vi "SUB_Chk_SWVer_MCS.vi"() -> (0 "SwVer_MCS":string, 1 "OK ?":bool)   [LabVIEW 2011]
uses:
  Instance           5 25Saved   SUB_Chk_SWVer_MCS .vi
  Instance           7 25Saved   SUB_Chk_SWVer_MCS .vi
  data/MCSDLL.dll
panel:
  out "Current Software Version":string
  out "UUT Model Type":string
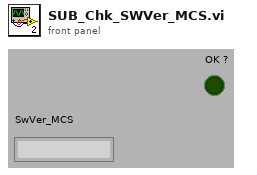
[diagram p1: front panel]
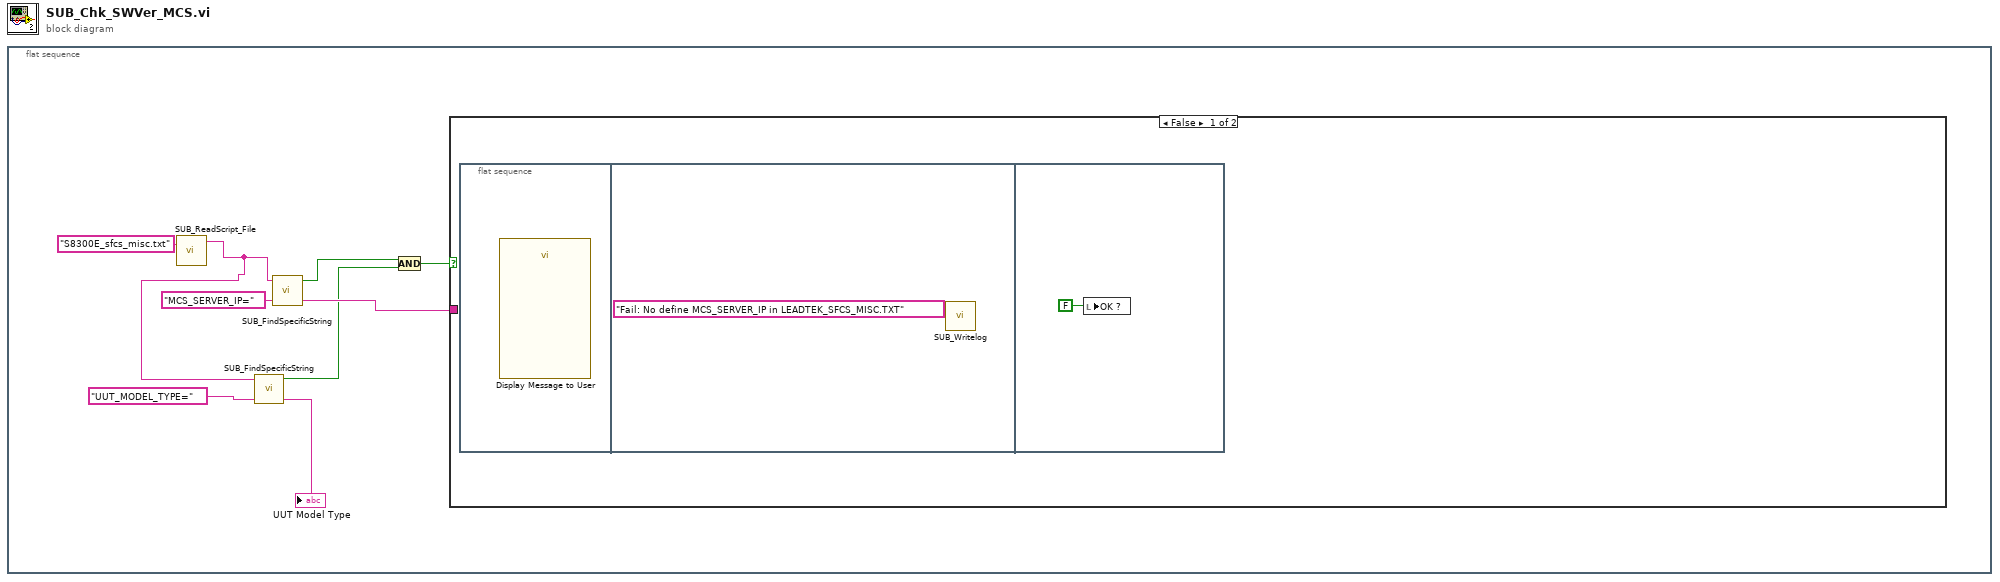
[diagram p0: block diagram]
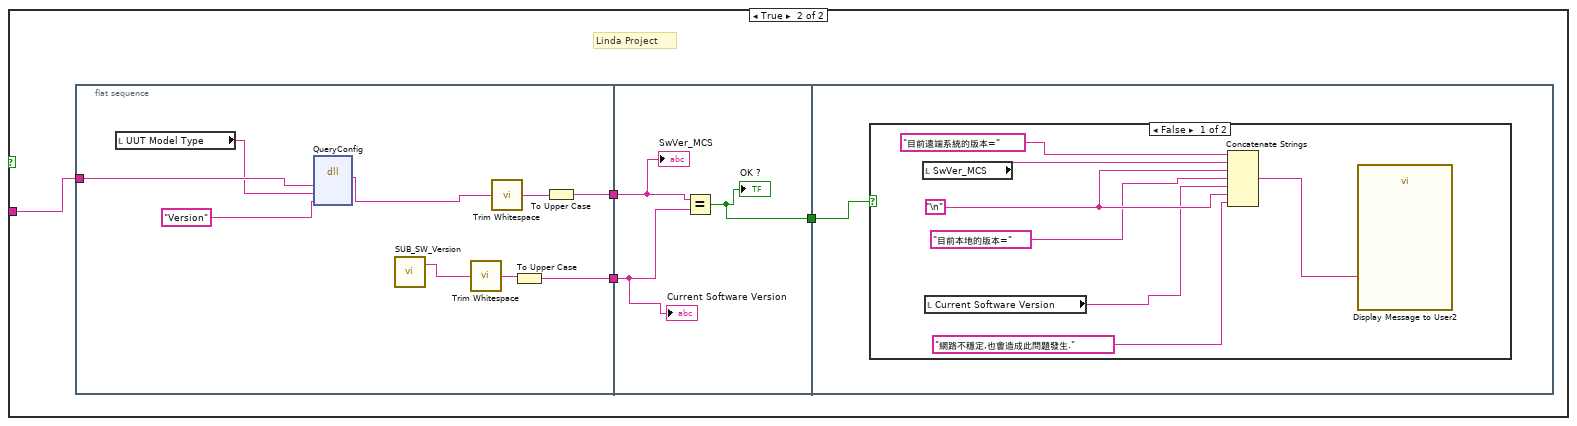
[diagram p2: hidden frame]
diagram:
  n1 = flat-sequence {
    frame #0 {
      n2 = call "SUB_ReadScript_File.vi"("Script FileName"="S8300E_sfcs_misc.txt") -> ("text"=w5:string)  [unwired: 1 in, 2 out]
      n3 = call "SUB_FindSpecificString.vi"("Find this String"="UUT_MODEL_TYPE=", "String data"=w5) -> ("before \"; \" string"=→"UUT Model Type":string, "Found"=w1:bool)  [unwired: 2 in]
      n4 = call "SUB_FindSpecificString.vi"("Find this String"="MCS_SERVER_IP=", "String data"=w5) -> ("before \"; \" string"=w7:string, "Found"=w2:bool)  [unwired: 2 in]
      n5 = And(x=w2, y=w1) -> (x .and. y?=w3:bool)
      n6 = case shown="False" w3 {
        tunnel: w7 -> [_ w15]
        frame False {
          n7 = flat-sequence {
            frame #0 {
              n8 = call "Display Message to User"() -> ()  [unwired: 10 in, 2 out]
            }
            frame #1 {
              n9 = call "SUB_Writelog.vi"("Pass/Fail"="Fail: No define MCS_SERVER_IP in LEADTEK_SFCS_MISC.TXT") -> ()  [unwired: 2 in]
            }
            frame #2 {
              n10 = local write "OK ?"(FALSE ("OK ?")) -> ()
            }
          }
        }
        frame True {
          # "Linda Project"
          n11 = flat-sequence {
            tunnel: w15 -> [w21]
            tunnel: [w17] -> w14
            tunnel: [w16] -> w13
            tunnel: w14 -> [w27]
            tunnel: w13 -> [w26]
            tunnel: [w25] -> w12
            tunnel: w12 -> [w28]
            frame #0 {
              n12 = local read "UUT Model Type"() -> (w20:string)
              n13 = dll-call lib="D:/S8300E_Project-current/data/MCSDLL.dll" fn="QueryConfig"("URL"=w21, "ProjectName"=w20, "CheckItem"="Version") -> (w23:string)  [unwired: 6 in, 2 out]
              n14 = call "SUB_SW_Version.vi"() -> ("Current Software Version"=w19:string)  [unwired: 3 in]
              n15 = call <vilib>:"Trim Whitespace.vi"("string"=w19) -> ("trimmed string"=w18:string)  [unwired: 1 in]
              n16 = call <vilib>:"Trim Whitespace.vi"("string"=w23) -> ("trimmed string"=w24:string)  [unwired: 1 in]
              n17 = To Upper Case(1:w18) -> (0:w16:string)
              n18 = To Upper Case(1:w24) -> (0:w17:string)
            }
            frame #1 {
              n19 = Equal?(x=w27, y=w26) -> (x = y?=w25:bool)
              "OK ?" <- w25
              "SwVer_MCS" <- w27
              "Current Software Version" <- w26
            }
            frame #2 {
              n20 = case shown="False" w28 {
                frame False {
                  w34 = "\n"
                  n21 = local read "SwVer_MCS"() -> (w31:string)
                  n22 = local read "Current Software Version"() -> (w33:string)
                  n23 = Concatenate Strings("目前遠端系統的版本=" ("string"), w31, w34, "目前本地的版本=" ("string"), w33, w34, "網路不穩定,也會造成此問題發生.") -> (w29:string)
                  n24 = call "Display Message to User2"("Message"=w29) -> ()  [unwired: 9 in, 2 out]
                }
                frame True {
                }
              }
            }
          }
        }
      }
    }
  }
